vi "oax_Build Device Info (DSA).vi"(9 "sample rate":dbl=1000.0 format="%0.2f", 11 "DSA device type":T1 items=["4472"=0, "4474"=10, "4461"=1, "4462"=11, "4464"=12, "449x"=6, "9232"=7, "9233"=2, "9234"=3, "9229"=4, "9239"=5]) -> (1 "device info":T2 {"DSA device type" items=["Custom"=0, "4472"=1, "4474"=11, "4461"=2, "4462"=12, "4464"=13, "449x"=7, "9232"=8, "9233"=3, "9234"=4, "9229"=5, "9239"=6]}, 3 "synchronization type":u16(ring) items=["by sharing sample clock", "by using reference clock"])   [LabVIEW 2017]
uses:
  <vilib>/addons/Sound and Vibration/Order Analysis/Example Support/sub VIs/OAXML_DSA Device Type.ctl
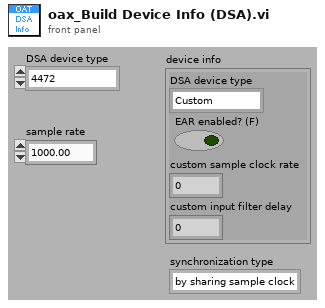
[diagram p1: front panel]
types:
  T1 = typedef "OAXML_DSA Device Type.ctl" = u16
  T2 = cluster{"DSA device type":u16, "EAR enabled? (F)":bool, "custom sample clock rate":dbl, "custom input filter delay":dbl}
  T3 = cluster{"device type":u16, "EAR enabled? (F)":bool, "custom sample clock rate":dbl, "custom input filter delay":dbl}
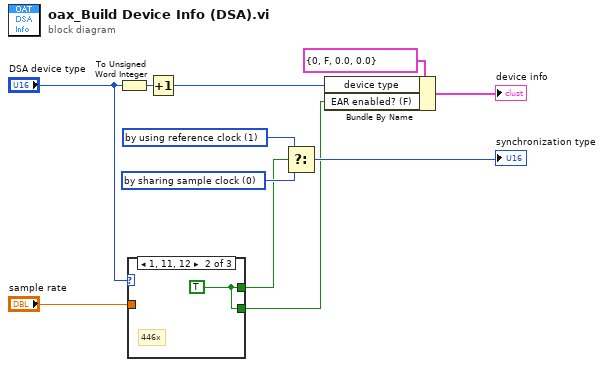
[diagram p0: block diagram]
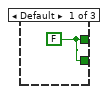
[diagram p2: hidden frame]
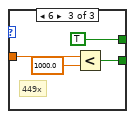
[diagram p3: hidden frame]
diagram:
  w7 = u16 0 items=["by sharing sample clock", "by using reference clock"] ("synchronization type")
  w8 = u16 1 items=["by sharing sample clock", "by using reference clock"] ("synchronization type")
  n1 = To Unsigned Word Integer(number="DSA device type") -> (unsigned 16bit integer=w1:T1)
  n2 = case shown="1, 11, 12" "DSA device type" {
    tunnel: [w12 w13 TRUE] -> w5
    tunnel: [w12 w13 w15] -> w4
    tunnel: "sample rate" -> [_ _ w16]
    frame Default {
      w12 = FALSE
    }
    frame 1, 11, 12 {
      w13 = TRUE
      # "446x"
    }
    frame 6 {
      # "449x"
      n3 = Less?(x=w16, y=1000.0) -> (x < y?=w15:bool)
    }
  }
  n4 = Increment(x=w1) -> (x+1=w10:T1)
  n5 = Select(t=w8, s=w5, f=w7) -> (s? t:f=→"synchronization type":u16)
  n6 = Bundle By Name(cluster=T3 {"device type"=0, "EAR enabled? (F)"=FALSE, "custom sample clock rate"=0.0, "custom input filter delay"=0.0} ("device info"), "device type"=w10, "EAR enabled? (F)"=w4) -> (→"device info":T3)
